vi "MHX Shell Heat Transfer Coefficient.vi"(6 "MHX Sec Pr":dbl, 7 "Sec Mass Flux":dbl, 9 "MHX Sec Phi":dbl, 10 "MHX Sec Re":dbl, 11 "Cp of FLiNaK":dbl) -> (3 "MHX Shell h":dbl)   [LabVIEW 2019]
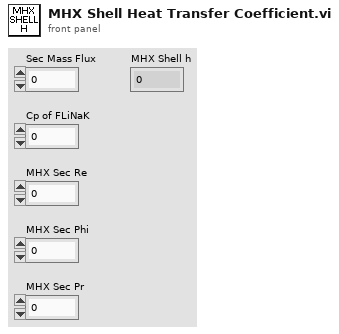
[diagram p1: front panel]
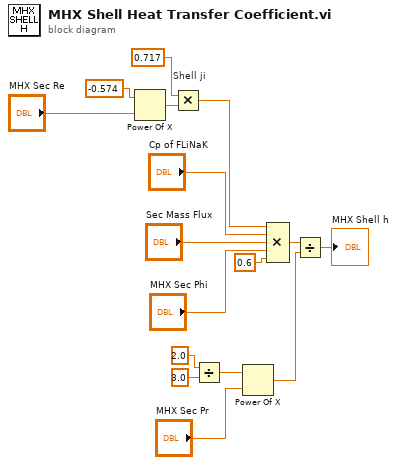
[diagram p0: block diagram]
diagram:
  n1 = Power Of X(1:"MHX Sec Re", 2:-0.574 ("y")) -> (0:w3:dbl)
  n2 = Multiply "Shell ji"(x=0.717, y=w3) -> (x*y=w5:dbl)
  n3 = Divide(x=2.0, y=3.0) -> (x/y=w12:dbl)
  n4 = Power Of X(1:"MHX Sec Pr", 2:w12) -> (0:w15:dbl)
  n5 = Compound Arithmetic op=MULTIPLY(w5, "Cp of FLiNaK", "Sec Mass Flux", "MHX Sec Phi", 0.6 ("value")) -> (w14:dbl)
  n6 = Divide(x=w14, y=w15) -> (x/y=→"MHX Shell h":dbl)
